vi "Keithley_IV_sendot_v2.vi"(0 "VISA resource name 2":refnum<visa-resource-name>="COM4", 1 "Waveform":i16(ring)=2 items=["Sin", "Cos", "Triang", "Square", "Saw Tooth", "Inc Ramp", "Dec Ramp", "White Noise"], 5 "N periods":dbl=3.0, 9 "dc offset":dbl format="%0.2f", 11 "Enable Voltage Source (F: Disable)":bool=TRUE, 12 "amplitude":dbl=1.0 format="%0.2f", 14 "N points/period":dbl=40.0) -> (3 "x*y":dbl, 4 "I-V":cluster{dbl[], dbl[]}(graph)={[0.0, 0.3090169943749474, 0.587785252292473, 0.8090169943749473, 0.9510565162951534, 1.0, 0.9510565162951535, 0.0, 0.0, 0.0, 0.0, 0.0, 0.0, 0.0, 0.0, 0.0, 0.0, 0.0, 0.0, 0.0, 0.0, 0.0, 0.0, 0.0, 0.0, 0.0, 0.0, 0.0, 0.0, 0.0, 0.0, 0.0, 0.0, 0.0, 0.0, 0.0, 0.0, 0.0, 0.0, 0.0, 0.0, 0.0, 0.0, 0.0, 0.0, 0.0, 0.0, 0.0, 0.0, 0.0, 0.0, 0.0, 0.0, 0.0, 0.0, 0.0, 0.0, 0.0, 0.0, 0.0, 0.0, 0.0, 0.0, 0.0, 0.0, 0.0, 0.0], [1133.576, 7749.111999999999, 15083.22, 20740.46, 23218.17, 24046.269999999997, 22248.17, 0.0, 0.0, 0.0, 0.0, 0.0, 0.0, 0.0, 0.0, 0.0, 0.0, 0.0, 0.0, 0.0, 0.0, 0.0, 0.0, 0.0, 0.0, 0.0, 0.0, 0.0, 0.0, 0.0, 0.0, 0.0, 0.0, 0.0, 0.0, 0.0, 0.0, 0.0, 0.0, 0.0, 0.0, 0.0, 0.0, 0.0, 0.0, 0.0, 0.0, 0.0, 0.0, 0.0, 0.0, 0.0, 0.0, 0.0, 0.0, 0.0, 0.0, 0.0, 0.0, 0.0, 0.0, 0.0, 0.0, 0.0, 0.0, 0.0, 0.0]}, 6 "Current":cluster{dbl[], dbl[]}(graph)={[-0.35771846771240234, 0.6306648254394531, 2.1383543014526367, 2.797945499420166, 3.454411029815674, 4.743261814117432, 5.399254322052002, 0.0, 0.0, 0.0, 0.0, 0.0, 0.0, 0.0, 0.0, 0.0, 0.0, 0.0, 0.0, 0.0, 0.0, 0.0, 0.0, 0.0, 0.0, 0.0, 0.0, 0.0, 0.0, 0.0, 0.0, 0.0, 0.0, 0.0, 0.0, 0.0, 0.0, 0.0, 0.0, 0.0, 0.0, 0.0, 0.0, 0.0, 0.0, 0.0, 0.0, 0.0, 0.0, 0.0, 0.0, 0.0, 0.0, 0.0, 0.0, 0.0, 0.0, 0.0, 0.0, 0.0, 0.0, 0.0, 0.0, 0.0, 0.0, 0.0, 0.0], [1133.576, 7749.111999999999, 15083.22, 20740.46, 23218.17, 24046.269999999997, 22248.17, 0.0, 0.0, 0.0, 0.0, 0.0, 0.0, 0.0, 0.0, 0.0, 0.0, 0.0, 0.0, 0.0, 0.0, 0.0, 0.0, 0.0, 0.0, 0.0, 0.0, 0.0, 0.0, 0.0, 0.0, 0.0, 0.0, 0.0, 0.0, 0.0, 0.0, 0.0, 0.0, 0.0, 0.0, 0.0, 0.0, 0.0, 0.0, 0.0, 0.0, 0.0, 0.0, 0.0, 0.0, 0.0, 0.0, 0.0, 0.0, 0.0, 0.0, 0.0, 0.0, 0.0, 0.0, 0.0, 0.0, 0.0, 0.0, 0.0, 0.0]}, 8 "Voltage":cluster{dbl[], dbl[]}(graph)={[-0.35771846771240234, 0.6306648254394531, 2.1383543014526367, 2.797945499420166, 3.454411029815674, 4.743261814117432, 5.399254322052002, 0.0, 0.0, 0.0, 0.0, 0.0, 0.0, 0.0, 0.0, 0.0, 0.0, 0.0, 0.0, 0.0, 0.0, 0.0, 0.0, 0.0, 0.0, 0.0, 0.0, 0.0, 0.0, 0.0, 0.0, 0.0, 0.0, 0.0, 0.0, 0.0, 0.0, 0.0, 0.0, 0.0, 0.0, 0.0, 0.0, 0.0, 0.0, 0.0, 0.0, 0.0, 0.0, 0.0, 0.0, 0.0, 0.0, 0.0, 0.0, 0.0, 0.0, 0.0, 0.0, 0.0, 0.0, 0.0, 0.0, 0.0, 0.0, 0.0, 0.0], [0.0, 0.3090169943749474, 0.587785252292473, 0.8090169943749473, 0.9510565162951534, 1.0, 0.9510565162951535, 0.0, 0.0, 0.0, 0.0, 0.0, 0.0, 0.0, 0.0, 0.0, 0.0, 0.0, 0.0, 0.0, 0.0, 0.0, 0.0, 0.0, 0.0, 0.0, 0.0, 0.0, 0.0, 0.0, 0.0, 0.0, 0.0, 0.0, 0.0, 0.0, 0.0, 0.0, 0.0, 0.0, 0.0, 0.0, 0.0, 0.0, 0.0, 0.0, 0.0, 0.0, 0.0, 0.0, 0.0, 0.0, 0.0, 0.0, 0.0, 0.0, 0.0, 0.0, 0.0, 0.0, 0.0, 0.0, 0.0, 0.0, 0.0, 0.0, 0.0]}, 10 "Appened output array":dbl[][](array[numeric]), 13 "Bool to sendot savineg":bool, 15 "x = y?":bool)   [LabVIEW 2021]
uses:
  <instrlib>/Keithley 648X Series/Keithley 648X Series.lvlib
  <vilib>/Analysis/NI_AALPro.lvlib
  <vilib>/Analysis/NI_AALBase.lvlib
panel:
  in  "Enable Zero Check (T: Enable)":bool=TRUE
  out "s? t:f":dbl
  out "App. Voltage":dbl
  in  "Weighting (Sample)":enum16{"Sample", "Population"}(ring)
  in  "Def redn SD":dbl=10.0 format="%#_13g"
  out "SD threshold":dbl
  out "Engineering string":string
  out "appended array":dbl[](array[numeric])
  out "Measurement":dbl
  in  "Range":dbl
  in  "duration":dbl=1.0 format="%0.2f"
  in  "Time Sample(ms)":u32=100
  in  "stop for KE":bool
  out "Current Waveform Chart":dbl[](graph)=[1133.576, 7749.111999999999, 15083.22, 20740.46, 23218.17, 24046.269999999997, 22248.17, 0.0, 0.0, 0.0, 0.0, 0.0, 0.0, 0.0, 0.0, 0.0, 0.0, 0.0, 0.0, 0.0, 0.0, 0.0, 0.0, 0.0, 0.0, 0.0, 0.0, 0.0, 0.0, 0.0, 0.0, 0.0, 0.0, 0.0, 0.0, 0.0, 0.0, 0.0, 0.0, 0.0, 0.0, 0.0, 0.0, 0.0, 0.0, 0.0, 0.0, 0.0, 0.0, 0.0, 0.0, 0.0, 0.0, 0.0, 0.0, 0.0, 0.0, 0.0, 0.0, 0.0, 0.0, 0.0, 0.0, 0.0, 0.0, 0.0, 0.0]
  in  "Autorange (T: Enable)":bool=TRUE
  out "?":dbl=5.399254322052002
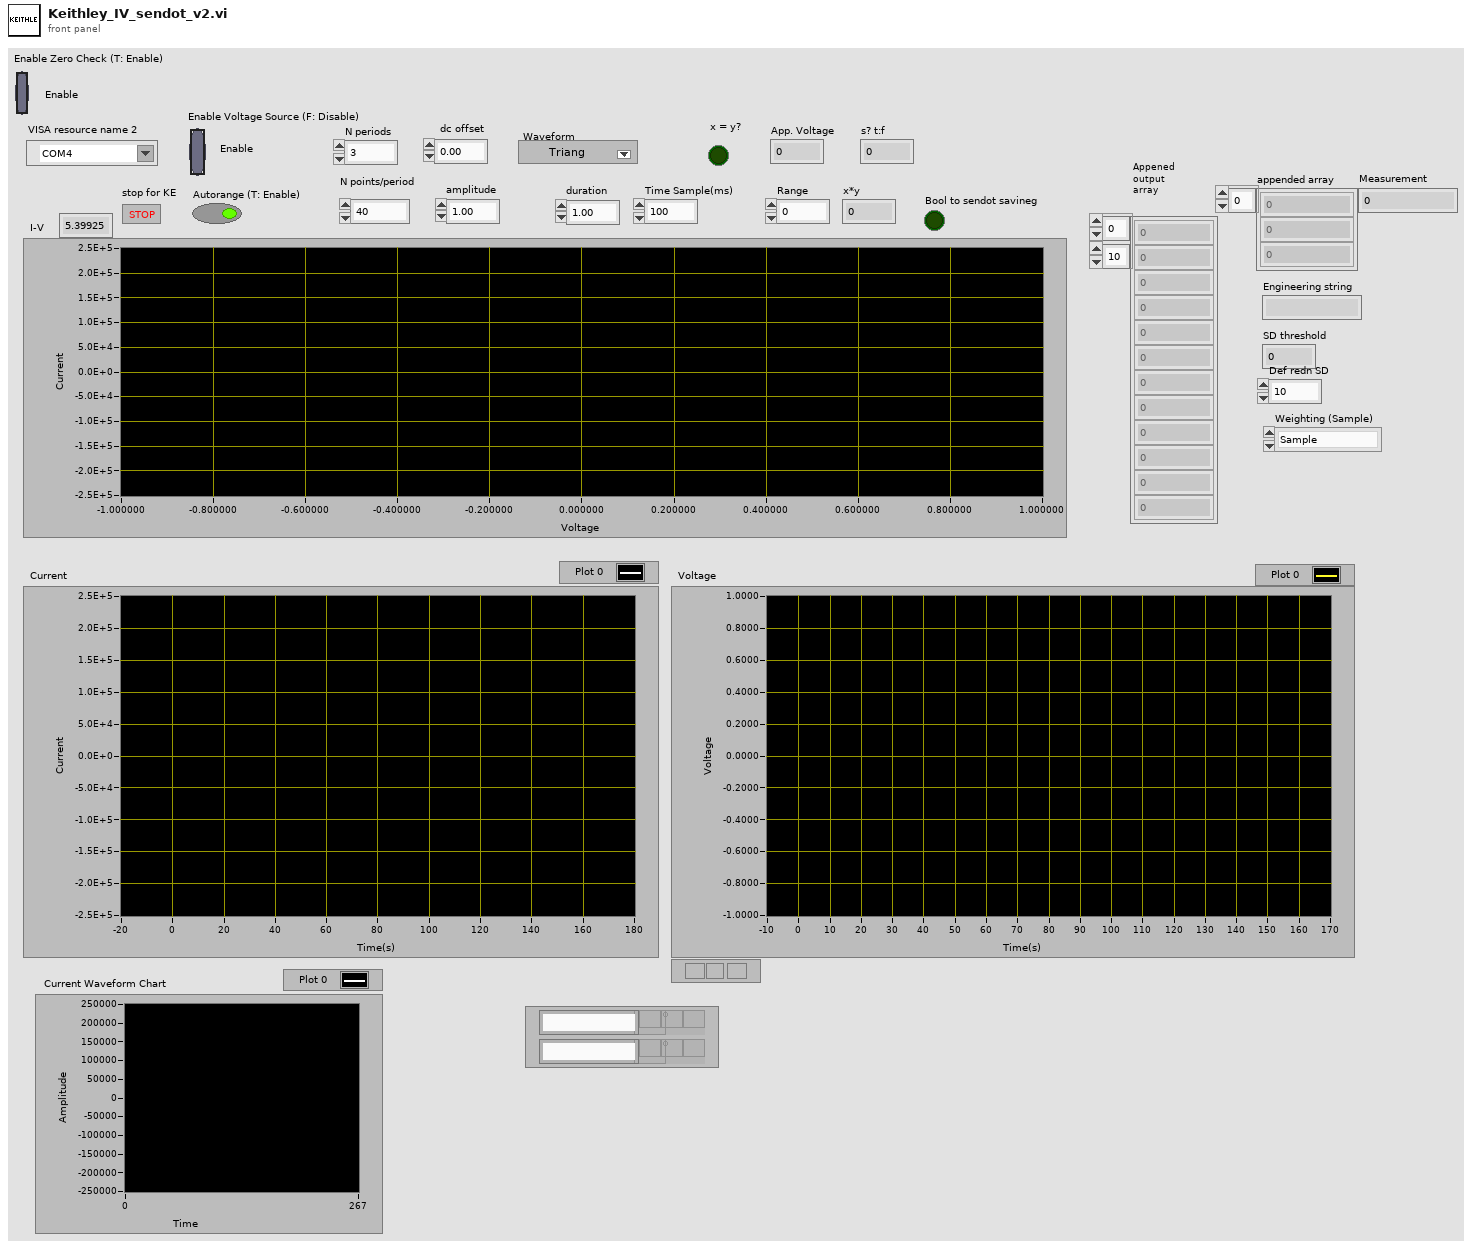
[diagram p1: front panel]
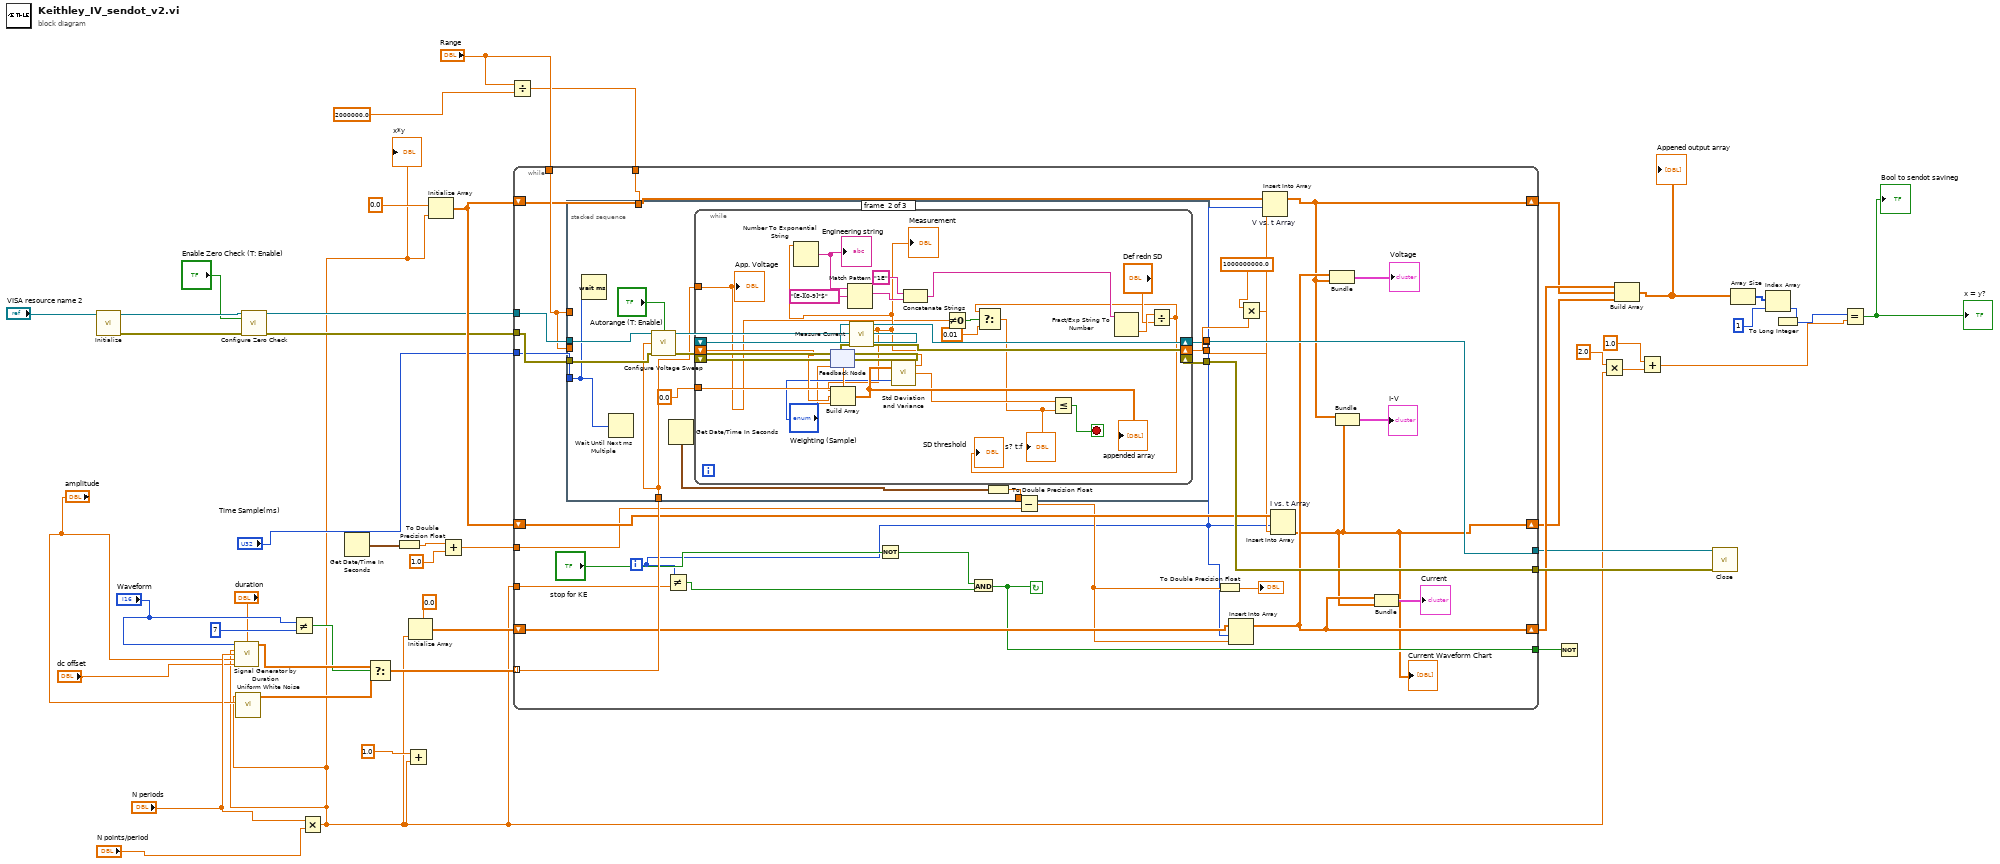
[diagram p0: block diagram]
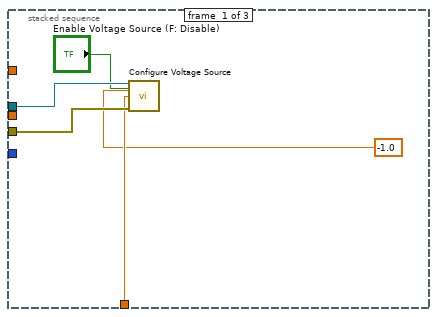
[diagram p2: hidden frame]
diagram:
  n1 = call <instrlib>:"Initialize.vi"("VISA resource name"="VISA resource name 2") -> ("error out"=w22:errorcluster, "VISA resource name out"=w20:refnum<visa-resource-name>)  [unwired: 9 in]
  n2 = call <instrlib>:"Configure Zero Check.vi"("VISA resource name"=w20, "Enable Zero Check (T: Enable)"="Enable Zero Check (T: Enable)", "error in (no error)"=w22) -> ("VISA resource name out"=w19:refnum<visa-resource-name>, "error out"=w21:errorcluster)  [unwired: 11 in]
  n3 = Not Equal?(x="Waveform", y=i16 7) -> (x != y?=w29:bool)
  n4 = Multiply(x="N periods", y="N points/period") -> (x*y=w2:dbl)
  "x*y" <- w2
  n5 = call <vilib>:"Signal Generator by Duration.vi"("signal type"="Waveform", "duration"="duration", "# of samples"=w2, "frequency"="N periods", "amplitude"="amplitude", "dc offset"="dc offset") -> ("signal"=w32:dbl[])  [unwired: 6 in, 3 out]
  n6 = call <vilib>:"Uniform White Noise.vi"("amplitude"="amplitude", "samples"=w2) -> ("uniform white noise"=w31:dbl[])  [unwired: 8 in, 1 out]
  n7 = Get Date/Time In Seconds() -> (seconds since 1Jan1904=w39:timestamp)
  n8 = Select(t=w32, s=w29, f=w31) -> (s? t:f=w44:dbl[])
  n9 = To Double Precision Float(number=w39) -> (double precision float=w35:dbl)
  n10 = Add(x=1.0, y=w2) -> ()  [unwired: 1 out]
  n11 = Initialize Array(0.0 ("element"), w2) -> (w42:dbl[])
  n12 = Initialize Array(0.0 ("element"), w2) -> (w38:dbl[])
  n13 = Add(x=w35, y=1.0) -> (x+y=w33:dbl)
  n14 = Divide(x="Range", y=2000000.0) -> (x/y=w23:dbl)
  n15 = while {
    tunnel: w19 -> [w78]
    tunnel: w21 -> [w77]
    tunnel: w44 -> [w76] mode=indexing
    tunnel: [w75] -> w43
    tunnel: [w74] -> w18
    tunnel: w2 -> [w72]
    tunnel: [w69] -> w40
    shift-right: [w56] -> w4
    shift-left: w38 -> [w49]
    shift-right: [w55] -> w3
    shift-left: w38 -> [w67]
    shift-right: [w66] -> w37
    shift-left: w42 -> [w73]
    tunnel: "Time Sample(ms)" -> [w62]
    tunnel: w33 -> [w61]
    tunnel: "Range" -> [w51]
    tunnel: w23 -> [w52]
    i -> [w50]
    stop <- w69 continue-if-true
    n16 = stacked-sequence {
      tunnel: w78 -> [w82 w93 _]
      tunnel: w77 -> [w83 w92 _]
      tunnel: w76 -> [w81 w84 w122]
      tunnel: [_ w87 _] -> w75
      tunnel: [_ w88 _] -> w74
      tunnel: [_ _ w122] -> w48
      tunnel: [_ w96 _] -> w65
      tunnel: w62 -> [_ w86 _]
      tunnel: [_ w95 _] -> w60
      tunnel: w51 -> [_ _ _]
      tunnel: w52 -> [_ _ _]
      tunnel: w51 -> [_ _ _]
      frame #0 {
        w79 = -1.0 items=["-1"=-1.0] ("Voltage Source Range")
        n17 = call <instrlib>:"Configure Voltage Source.vi"("VISA resource name"=w82, "Enable Voltage Source (F: Disable)"="Enable Voltage Source (F: Disable)", "Voltage Source Range (10 V)"=w79, "Voltage Level (0 V)"=w81, "error in (no error)"=w83) -> ()  [unwired: 9 in, 2 out]
      }
      frame #1 {
        n18 = Wait (ms)(milliseconds to wait=w86) -> ()  [unwired: 1 out]
        n19 = Wait Until Next ms Multiple(millisecond multiple=w86) -> ()  [unwired: 1 out]
        n20 = call <instrlib>:"Configure Voltage Sweep.vi"("VISA resource name"=w93, "Autoconfig Arm (T: Enable)"="Autorange (T: Enable)", "Voltage Sweep Stop (10V)"=w84, "error in (no error)"=w92) -> ("VISA resource name out"=w90:refnum<visa-resource-name>, "error out"=w91:errorcluster)  [unwired: 10 in]
        n21 = Get Date/Time In Seconds() -> (seconds since 1Jan1904=w94:timestamp)
        n22 = while {
          shift-right: [w118] -> w87
          shift-left: w91 -> [w121]
          shift-right: [w119] -> w88
          shift-left: w90 -> [w120]
          shift-right: [w105] -> w96
          shift-left: _ -> [w113]
          tunnel: 0.0 ("mean") -> [w114]
          tunnel: w84 -> [w101]
          stop <- w117 stop-if-true
          n23 = feedback #1(w114) -> (w111:dbl)
          n24 = call <instrlib>:"Measure Current.vi"("VISA resource name"=w120, "error in (no error)"=w121) -> ("VISA resource name out"=w119:refnum<visa-resource-name>, "Measurement"=w105:dbl, "error out"=w118:errorcluster)  [unwired: 11 in]
          "Measurement" <- w105
          n25 = Number To Exponential String(number=w105) -> (E-format string=w110:string)  [unwired: 3 in]
          "Engineering string" <- w110
          n26 = Build Array(w105, w113, w111) -> (w116:dbl[])
          "appended array" <- w116
          n27 = Match Pattern(string=w110, regular expression="[E-][0-9]*$") -> (match substring=w107:string)  [unwired: 1 in, 3 out]
          n28 = call <vilib>:"Std Deviation and Variance.vi"("X"=w116, "Weighting (Sample)"="Weighting (Sample)") -> ("mean"=w102:dbl, "standard deviation"=w115:dbl)  [unwired: 1 out]
          n29 = feedback-in #1(w102) -> ()
          n30 = Concatenate Strings("1E" ("string"), w107) -> (w106:string)
          n31 = Not Equal To 0?(x=w101) -> (x != 0?=w100:bool)
          n32 = Fract/Exp String To Number(string=w106) -> (number=w104:dbl)  [unwired: 3 in, 1 out]
          n33 = Divide(x=w104, y="Def redn SD") -> (x/y=w99:dbl)
          "SD threshold" <- w99
          n34 = Select(t=w99, s=w100, f=0.01) -> (s? t:f=w98:dbl)
          "s? t:f" <- w98
          n35 = Less Or Equal?(x=w115, y=w98) -> (x <= y?=w117:bool)
          "App. Voltage" <- w101
        }
        n36 = To Double Precision Float(number=w94) -> (double precision float=w95:dbl)
      }
      frame #2 {
      }
    }
    n37 = Not Equal?(x=w50, y=w72) -> (x != y?=w71:bool)
    n38 = Not(x="stop for KE") -> (.not. x?=w70:bool)
    n39 = And(x=w70, y=w71) -> (x .and. y?=w69:bool)
    n40 = Subtract(x=w60, y=w61) -> (x-y=w59:dbl)
    n41 = To Double Precision Float(number=w59) -> (double precision float=→"?":dbl)
    n42 = Insert Into Array(array=w73, index=w50, new element=w59) -> (w66:dbl[])
    n43 = Multiply(x=1000000000.0, y=w65) -> (x*y=w63:dbl)
    n44 = Insert Into Array "V vs. t Array"(array=w49, index=w50, new element=w48) -> (w56:dbl[])
    n45 = Insert Into Array "I vs. t Array"(array=w67, index=w50, new element=w63) -> (w55:dbl[])
    "Current Waveform Chart" <- w55
    n46 = Bundle(w66, w56) -> (→"Voltage":cluster{dbl[], dbl[]})  [unwired: 1 in]
    n47 = Bundle(w56, w55) -> (→"I-V":cluster{dbl[], dbl[]})  [unwired: 1 in]
    n48 = Bundle(w66, w55) -> (→"Current":cluster{dbl[], dbl[]})  [unwired: 1 in]
  }
  n49 = Not(x=w40) -> ()  [unwired: 1 out]
  n50 = Multiply(x=2.0, y=w2) -> (x*y=w17:dbl)
  n51 = Build Array(w37, w4, w3) -> (w8:dbl[][])
  "Appened output array" <- w8
  n52 = Add(x=1.0, y=w17) -> (x+y=w14:dbl)
  n53 = call <instrlib>:"Close.vi"("error in (no error)"=w43, "VISA resource name"=w18) -> ()  [unwired: 9 in, 1 out]
  n54 = Array Size(array=w8) -> (size(s)=w13:i32[])
  n55 = Index Array(array=w13, index=1) -> (element=w11:i32)
  n56 = To Long Integer(number=w11) -> (32bit integer=w10:i32)
  n57 = Equal?(x=w10, y=w14) -> (x = y?=→"x = y?" →"Bool to sendot savineg":bool)
